vi "ABC2DQ.vi"(0 "ABC":waveform(dbl)[](array[waveform]), 1 "Waveform Name":string) -> (2 "d":waveform(dbl), 3 "q":waveform(dbl), 4 "Park Vector ^2":waveform(dbl))   [LabVIEW 2020]
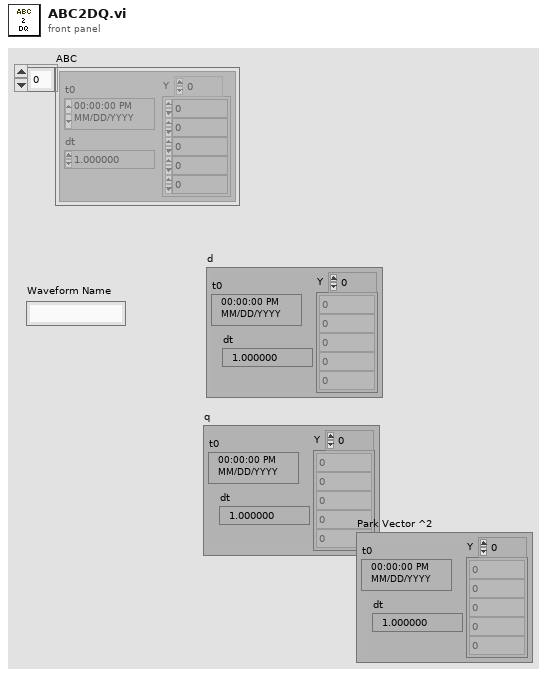
[diagram p1: front panel]
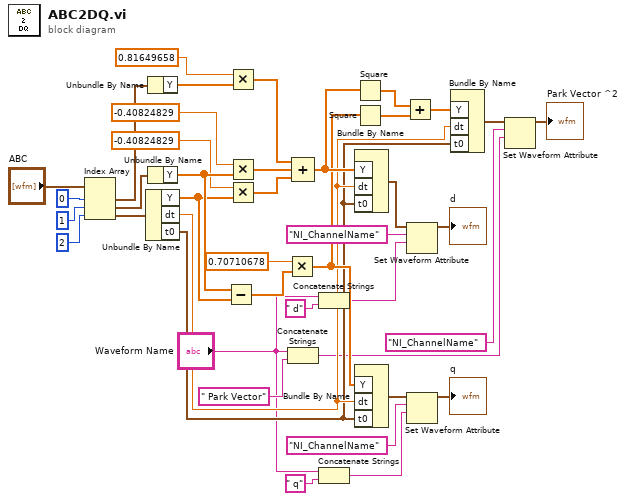
[diagram p0: block diagram]
diagram:
  n1 = Index Array(array="ABC", index #1=0 ("index"), index #2=1 ("index"), index #3=2 ("index")) -> (element #1=w37:waveform(dbl), element #2=w36:waveform(dbl), element #3=w35:waveform(dbl))
  n2 = Unbundle By Name(w35) -> ("Y"=w26:dbl[], "dt"=w18:dbl, "t0"=w17:timestamp)
  n3 = Unbundle By Name(w37) -> ("Y"=w33:dbl[])
  n4 = Unbundle By Name(w36) -> ("Y"=w27:dbl[])
  n5 = Subtract(x=w27, y=w26) -> (x-y=w25:dbl[])
  n6 = Multiply(x=0.81649658, y=w33) -> (x*y=w31:dbl[])
  n7 = Multiply(x=-0.40824829, y=w27) -> (x*y=w30:dbl[])
  n8 = Multiply(x=-0.40824829, y=w26) -> (x*y=w29:dbl[])
  n9 = Multiply(x=0.70710678, y=w25) -> (x*y=w22:dbl[])
  n10 = Concatenate Strings("Waveform Name", " Park Vector" ("string")) -> (w12:string)
  n11 = Compound Arithmetic op=ADD(w31, w30, w29) -> (w23:dbl[])
  n12 = Concatenate Strings("Waveform Name", " d" ("string")) -> (w9:string)
  n13 = Concatenate Strings("Waveform Name", " q" ("string")) -> (w6:string)
  n14 = Square(x=w23) -> (x^2=w21:dbl[])
  n15 = Square(x=w22) -> (x^2=w20:dbl[])
  n16 = Bundle By Name("Y"=w23, "dt"=w18, "t0"=w17) -> (w8:waveform(dbl))  [unwired: 1 in]
  n17 = Bundle By Name("Y"=w22, "dt"=w18, "t0"=w17) -> (w2:waveform(dbl))  [unwired: 1 in]
  n18 = Add(x=w21, y=w20) -> (x+y=w19:dbl[])
  n19 = Set Waveform Attribute(5:w9, 6:"NI_ChannelName" ("name"), 7:w8) -> (3:→"d":waveform(dbl))  [unwired: 1 in, 2 out]
  n20 = Set Waveform Attribute(5:w6, 6:"NI_ChannelName" ("name"), 7:w2) -> (3:→"q":waveform(dbl))  [unwired: 1 in, 2 out]
  n21 = Bundle By Name("Y"=w19, "dt"=w18, "t0"=w17) -> (w16:waveform(dbl))  [unwired: 1 in]
  n22 = Set Waveform Attribute(5:w12, 6:"NI_ChannelName" ("name"), 7:w16) -> (3:→"Park Vector ^2":waveform(dbl))  [unwired: 1 in, 2 out]
